vi "Change Controls.vi"(7 "Adjust All?":bool, 8 "Indicators":string[][](array[string]), 9 "Controls":string[][](array[string]), 10 "VI Index":i32, 11 "VI Data":T1[](array[typedef])) -> (3 "VI Data out":T1[](array[typedef]))   [LabVIEW 2023, in "VI Properties Editor.lvlib"]
uses:
  VI Properties Editor.lvlib
  CTLs/VI Data.ctl
  <vilib>/picture/picture.llb/imagedata.ctl
  CTLs/VI Properties.ctl
  CTLs/Control Properties.ctl
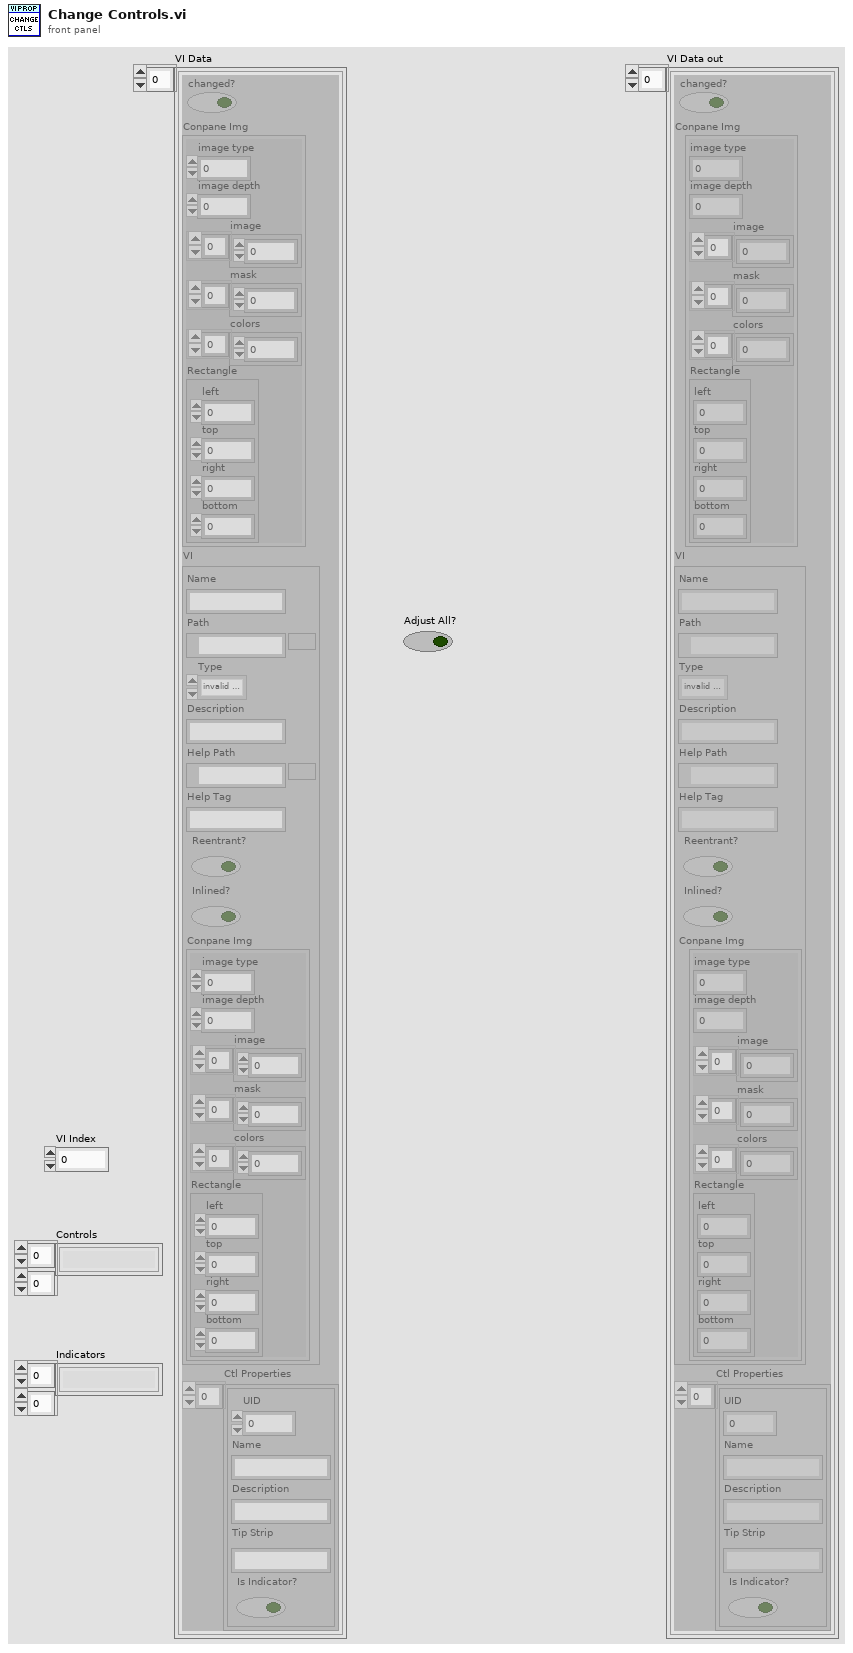
[diagram p1: front panel]
types:
  T1 = typedef "VI Properties Editor.lvlib/VI Data.ctl" = cluster{"changed?":bool, "Conpane Img":T2, "VI":T3, "Ctl Properties":T4[]}
  T2 = typedef "imagedata.ctl" = cluster{"image type":i32, "image depth":i32, "image":u8[], "mask":u8[], "colors":u32[], "Rectangle":cluster{"left":i16, "top":i16, "right":i16, "bottom":i16}}
  T3 = typedef "VI Properties Editor.lvlib/VI Properties.ctl" = cluster{"Name":string, "Path":path, "Type":enum32{"invalid VI type", "Standard VI", "Control VI", "Global VI", "Polymorphic VI", "Configuration VI", "SubSystem", "Facade VI", "Method VI", "Statechart Diagram VI"}, "Description":string, "Help Path":path, "Help Tag":string, "Reentrant?":bool, "Inlined?":bool, "Conpane Img":T2}
  T4 = typedef "VI Properties Editor.lvlib/Control Properties.ctl" = cluster{"UID":i32, "Name":string, "Description":string, "Tip Strip":string, "Is Indicator?":bool}
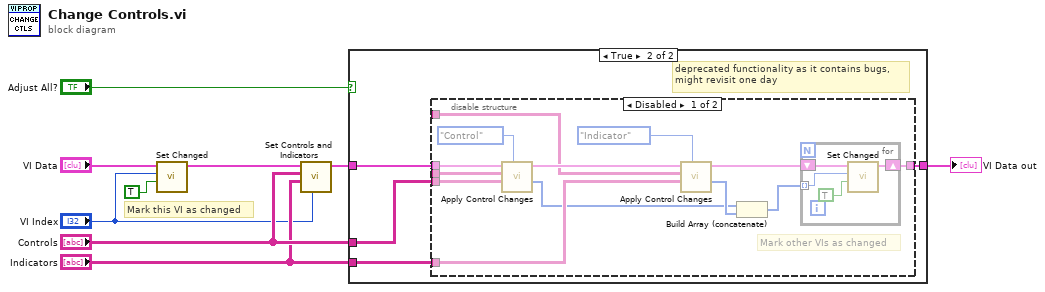
[diagram p0: block diagram]
diagram:
  # "Mark this VI as changed"
  n1 = call "Set Changed.vi"("Changed?"=TRUE ("changed?"), "VI Index"="VI Index", "VI Data in"="VI Data") -> ("VI Data out"=w7:T1[])  [unwired: 8 in]
  n2 = call "Set Controls and Indicators.vi"("VI Index"="VI Index", "Indicators"="Indicators", "Controls"="Controls", "VI Data In"=w7) -> ("VI Data Out"=w9:T1[])  [unwired: 7 in]
  n3 = case shown="True" "Adjust All?" {
    tunnel: "Controls" -> [_ w13]
    tunnel: "Indicators" -> [_ w12]
    tunnel: w9 -> [w10 w14]
    tunnel: [w10 w11] -> w3
    frame False {
    }
    frame True {
      # "deprecated functionality as it contains bugs,\nmight revisit one day"
      n4 = disable-structure shown="Disabled" {
        disable-tunnel: w14 -> [w27 w32]
        disable-tunnel: _ -> [w25 _]
        disable-tunnel: w13 -> [w24 _]
        disable-tunnel: _ -> [w23 _]
        disable-tunnel: w12 -> [w22 _]
        disable-tunnel: [w20 w32] -> w11
        frame Disabled {
          # "Mark other VIs as changed"
          n5 = call "Apply Control Changes.vi"("Type"=enum16{"Control", "Indicator"}."Control", "New"=w24, "Old"=w25, "Data In"=w27) -> ("Changed Indices"=w15:i32[], "Data Out"=w26:T1[])  [unwired: 6 in]
          n6 = call "Apply Control Changes.vi"("Type"=enum16{"Control", "Indicator"}."Indicator", "New"=w22, "Old"=w23, "Data In"=w26) -> ("Changed Indices"=w21:i32[], "Data Out"=w18:T1[])  [unwired: 6 in]
          n7 = Build Array (concatenate)(w15, w21) -> (w19:i32[])
          n8 = for {
            shift-right: [w30] -> w20
            shift-left: w18 -> [w31]
            tunnel: w19 -> [w29] mode=indexing
            n9 = call "Set Changed.vi"("Changed?"=TRUE ("new element/subarray"), "VI Index"=w29, "VI Data in"=w31) -> ("VI Data out"=w30:T1[])  [unwired: 8 in]
          }
        }
        frame Enabled {
        }
      }
    }
  }
  "VI Data out" <- w3
